vi "SetMode.vi"(2 "State":bool, 3 "Mode":T1(ring), 4 "Device":u8=1, 5 "Serial port":refnum<visa-resource-name>) -> (0 "Device out":u8=1, 1 "Serial port out":refnum<visa-resource-name>)   [LabVIEW 2021]
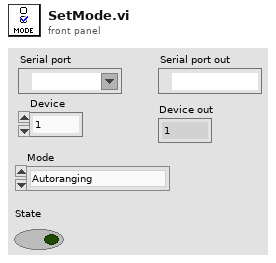
[diagram p1: front panel]
types:
  T1 = enum16{"Autoranging", "4 wire mode", "Guard mode", "Thermal control"}
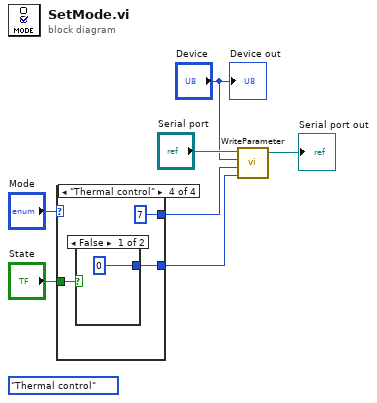
[diagram p0: block diagram]
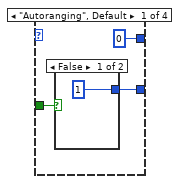
[diagram p2: hidden frame]
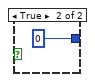
[diagram p3: hidden frame]
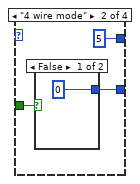
[diagram p4: hidden frame]
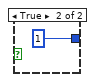
[diagram p5: hidden frame]
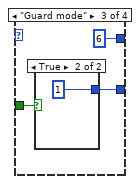
[diagram p6: hidden frame]
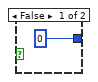
[diagram p7: hidden frame]
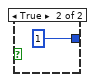
[diagram p8: hidden frame]
diagram:
  (unwired) T1."Thermal control"
  n1 = case shown="\"Thermal control\"" "Mode" {
    tunnel: "State" -> [w9 w14 w19 w25]
    tunnel: [u32 0 u32 5 u32 6 u32 7] -> w3
    tunnel: [w8 w13 w18 w24] -> w2
    frame "Autoranging", Default {
      n2 = case shown="False" w9 {
        tunnel: [1 0] -> w8
        frame False {
        }
        frame True {
        }
      }
    }
    frame "4 wire mode" {
      n3 = case shown="False" w14 {
        tunnel: [0 1] -> w13
        frame False {
        }
        frame True {
        }
      }
    }
    frame "Guard mode" {
      n4 = case shown="True" w19 {
        tunnel: [0 1] -> w18
        frame False {
        }
        frame True {
        }
      }
    }
    frame "Thermal control" {
      n5 = case shown="False" w25 {
        tunnel: [0 1] -> w24
        frame False {
        }
        frame True {
        }
      }
    }
  }
  n6 = call "WriteParameter.vi"("Value"=w2, "Address"=w3, "Device"="Device", "Serial port"="Serial port") -> ("Serial port out"=→"Serial port out":refnum<visa-resource-name>)  [unwired: 2 in]
  "Device out" <- "Device"
